vi "Send Message.vi"(6 "ID":string, 8 "error in (no error)":errorcluster, 9 "Data":variant, 10 "Command":string, 11 "RemoteControl in":refnum<class "RemoteControl.lvclass">) -> (0 "error out":errorcluster, 3 "RemoteControl out":refnum<class "RemoteControl.lvclass">)   [LabVIEW 2019, in "RemoteControl.lvlib" / "RemoteControl.lvclass"]
uses:
  RemoteControl.lvclass
  Typedefs/Message--Cluster.ctl
  RemoteControl.lvclass/RemoteControl.ctl
  Private/RemoteControl.GlobalVariable.vi
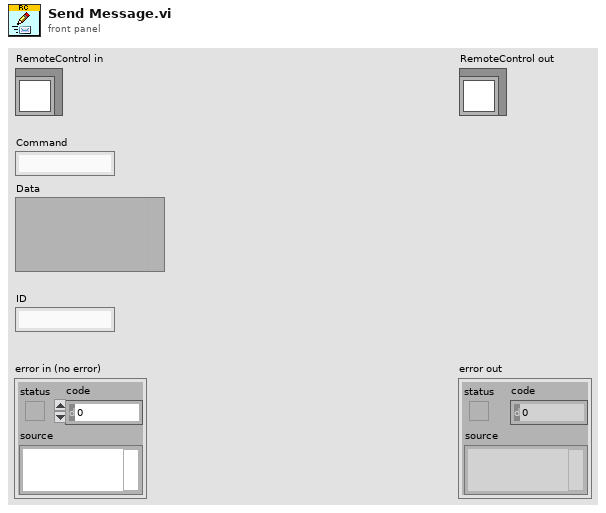
[diagram p1: front panel]
types:
  T1 = typedef "RemoteControl.lvlib/RemoteControl.lvclass/Message--Cluster.ctl" = cluster{"Command":string, "Data":variant, "ID":string}
  T2 = typedef "RemoteControl.lvlib/RemoteControl.lvclass/RC Process Type--Enum.ctl" = enum16{"Listener", "Server", "Client"}
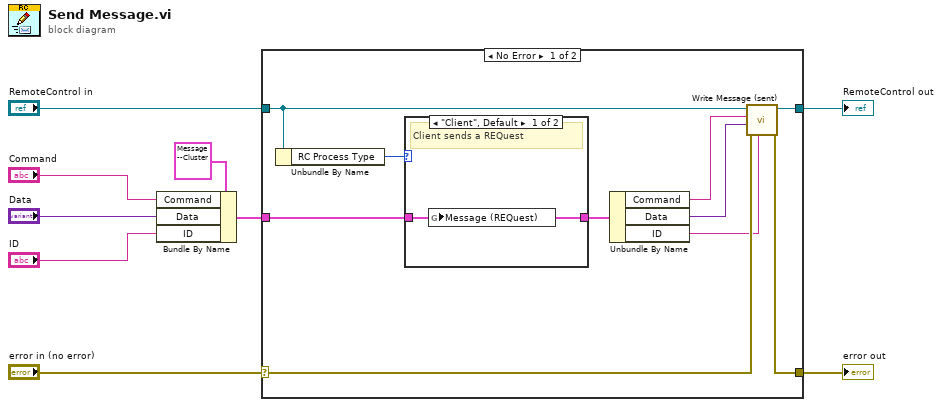
[diagram p0: block diagram]
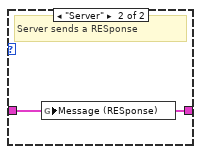
[diagram p2: hidden frame]
diagram:
  n1 = Bundle By Name(cluster=T1 {"Command"="", "Data"=variant(string ""), "ID"=""} ("Message"), "Command"="Command", "Data"="Data", "ID"="ID") -> (w6:T1)
  n2 = case shown="No Error" "error in (no error)" {
    selector: "error in (no error)" -> [w18 w23]
    tunnel: [w17 w23] -> w9
    tunnel: [w19 w22] -> w7
    tunnel: "RemoteControl in" -> [w12 w22]
    tunnel: w6 -> [w16 _]
    frame No Error {
      n3 = Unbundle By Name(w12) -> ("RC Process Type"=w11:T2)
      n4 = case shown="\"Client\", Default" w11 {
        tunnel: w16 -> [w20 w21]
        tunnel: [w20 w21] -> w10
        frame "Client", Default {
          # "Client sends a REQuest"
          n5 = global write "RemoteControl.GlobalVariable.vi" "Message (REQuest)"(w20) -> ()
        }
        frame "Server" {
          # "Server sends a RESponse"
          n6 = global write "RemoteControl.GlobalVariable.vi" "Message (RESponse)"(w21) -> ()
        }
      }
      n7 = Unbundle By Name(w10) -> ("Command"=w15:string, "Data"=w14:variant, "ID"=w13:string)
      n8 = call "Write Message (sent).vi"("ID (sent)"=w13, "error in (no error)"=w18, "Data"=w14, "Command (sent)"=w15, "RemoteControl in"=w12) -> ("error out"=w17:errorcluster, "RemoteControl out"=w19:refnum<class "RemoteControl.lvclass">)  [unwired: 5 in]
    }
    frame Error {
    }
  }
  "error out" <- w9
  "RemoteControl out" <- w7
